vi "PNS Grenzwerte pruefen.vi"(8 "Option":bool, 9 "Wert":dbl, 11 "Parameternamen PNS":T1=enum."Heizkreis 3") -> (0 "AbschMax":bool, 1 "AbschMin":bool, 2 "WarnMax":bool, 3 "WarnMin":bool, 4 "Regler":u16, 5 "F.Br.":bool)   [LabVIEW 2020, in "PNS.lvlib"]
uses:
  PNS.lvlib
  Parameternamen PNS.ctl
  Aktionen FGV Grenzwerte.ctl
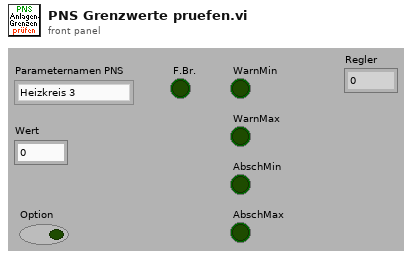
[diagram p1: front panel]
types:
  T1 = typedef "PNS.lvlib/Parameternamen PNS.ctl" = enum16{"Heizkreis 1", "Heizkreis 2", "Heizkreis 3", "Heizkreis 4", "Heizkreis 5", "Heizkreis 6", "Heizkreis 7", "Heizkreis 8"}
  T2 = typedef "PNS.lvlib/Aktionen FGV Grenzwerte.ctl" = enum16{"lesen", "Grenzw. schreiben", "Anweisungscode", "IP-Adresse", "laden", "speichern", "Anweisungscode vorgeben"}
  T3 = typedef "Steuerung PNS.lvclass/Anlegengrenzwerte PNS.ctl" = cluster{"Filter:":T4, "Ventilplatte:":T4, "Heizleitung 1:":T4, "Heizleitung 2:":T4, "Heizleitung 3:":T4, "Heizleitung 4:":T4, "Heizleitung 5:":T4, "Heizleitung 6:":T4}
  T4 = typedef "Steuerung PNS.lvclass/Anlagengrenzwerte Parameteranzeige.ctl" = cluster{"Sollwert":T5, "Warn-Min":T5, "Warn-Max":T5, "Abschalt-Min":T5, "Abschalt-Max":T5, "Regler":u16, "AnlagenParameter":string}
  T5 = typedef "Zahlen-Eingabefeld.ctl" = sgl
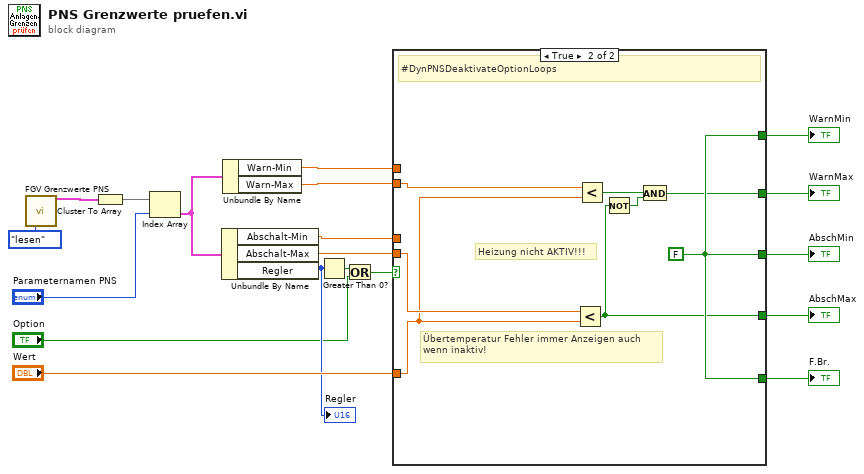
[diagram p0: block diagram]
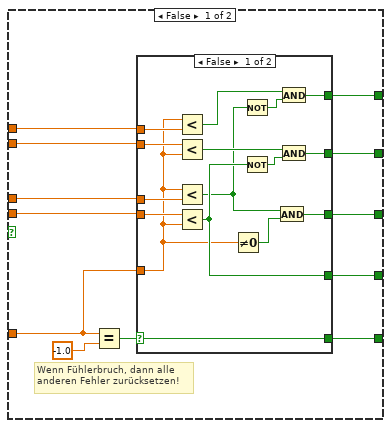
[diagram p2: hidden frame]
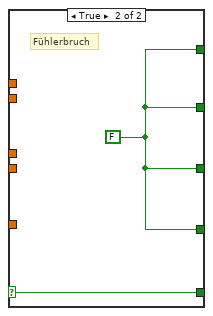
[diagram p3: hidden frame]
diagram:
  n1 = call "FGV Grenzwerte PNS.vi"("Aktionen FGV Grenzwerte"=Aktionen_FGV_Grenzwerte."lesen") -> ("Grenzwerte PNS 2"=w6:T3)  [unwired: 12 in, 2 out]
  n2 = Cluster To Array(cluster=w6) -> (array=w19:T4[])
  n3 = Index Array(array=w19, index="Parameternamen PNS") -> (element=w18:T4)
  n4 = Unbundle By Name(w18) -> ("Abschalt-Min"=w15:T5, "Abschalt-Max"=w14:T5, "Regler"=w4:u16)
  "Regler" <- w4
  n5 = Unbundle By Name(w18) -> ("Warn-Min"=w17:T5, "Warn-Max"=w16:T5)
  n6 = Greater Than 0?(x=w4) -> (x > 0?=w3:bool)
  n7 = Or(x=w3, y="Option") -> (x .or. y?=w2:bool)
  n8 = case shown="True" w2 {
    tunnel: w17 -> [w31 _]
    tunnel: w16 -> [w30 w50]
    tunnel: w15 -> [w29 _]
    tunnel: w14 -> [w28 w56]
    tunnel: [w27 w57] -> w13
    tunnel: [w26 w52] -> w12
    tunnel: [w25 w57] -> w11
    tunnel: [w24 w53] -> w10
    tunnel: [w23 w57] -> w9
    tunnel: "Wert" -> [w22 w51]
    frame False {
      # "Wenn Fühlerbruch, dann alle \nanderen Fehler zurücksetzen!"
      n9 = Equal?(x=w22, y=-1.0) -> (x = y?=w21:bool)
      n10 = case shown="False" w21 {
        selector: w21 -> [w36 w49]
        tunnel: w31 -> [w47 _]
        tunnel: w30 -> [w46 _]
        tunnel: w29 -> [w45 _]
        tunnel: w28 -> [w44 _]
        tunnel: [w39 w48] -> w23
        tunnel: [w38 w48] -> w24
        tunnel: [w32 w48] -> w25
        tunnel: [w37 w48] -> w26
        tunnel: w22 -> [w35 _]
        tunnel: [w36 w49] -> w27
        frame False {
          n11 = Less?(x=w35, y=w47) -> (x < y?=w43:bool)
          n12 = Less?(x=w46, y=w35) -> (x < y?=w40:bool)
          n13 = Less?(x=w35, y=w45) -> (x < y?=w33:bool)
          n14 = Less?(x=w44, y=w35) -> (x < y?=w37:bool)
          n15 = Not Equal To 0?(x=w35) -> (x != 0?=w34:bool)
          n16 = Not(x=w33) -> (.not. x?=w42:bool)
          n17 = Not(x=w37) -> (.not. x?=w41:bool)
          n18 = And(x=w33, y=w34) -> (x .and. y?=w32:bool)
          n19 = And(x=w43, y=w42) -> (x .and. y?=w39:bool)
          n20 = And(x=w40, y=w41) -> (x .and. y?=w38:bool)
        }
        frame True {
          w48 = FALSE
          # "Fühlerbruch"
        }
      }
    }
    frame True {
      w57 = FALSE
      # "Übertemperatur Fehler immer Anzeigen auch\nwenn inaktiv!"
      # "Heizung nicht AKTIV!!!"
      # "#DynPNSDeaktivateOptionLoops"
      n21 = Less?(x=w56, y=w51) -> (x < y?=w52:bool)
      n22 = Less?(x=w50, y=w51) -> (x < y?=w55:bool)
      n23 = Not(x=w52) -> (.not. x?=w54:bool)
      n24 = And(x=w55, y=w54) -> (x .and. y?=w53:bool)
    }
  }
  "WarnMin" <- w9
  "WarnMax" <- w10
  "AbschMin" <- w11
  "AbschMax" <- w12
  "F.Br." <- w13
